vi "Initiate Pulse Test.vi"(7 "Timeout (10000 ms)":u32=10000, 8 "error in":errorcluster, 10 "Tag":u32=1, 11 "VISA resource name":refnum<visa-resource-name>) -> (0 "error out":errorcluster, 1 "Message":string, 2 "Success":bool, 3 "VISA resource name out":refnum<visa-resource-name>, 4 "Command String":string)   [LabVIEW 2012, in "Keithley 2600 Series.lvlib"]
doc: "This VI will instruct the instrument to initiate the output of a pre-configured pulse train.\n\n<b>Functions and Attributes Used</b>\nInititatePulseTest(tag)"
uses:
  Keithley 2600 Series.lvlib
  Private/GlobalVariables.vi
panel:
  # "(c) 2008 Keithley Instruments, Inc.  ALL RIGHTS RESERVED."
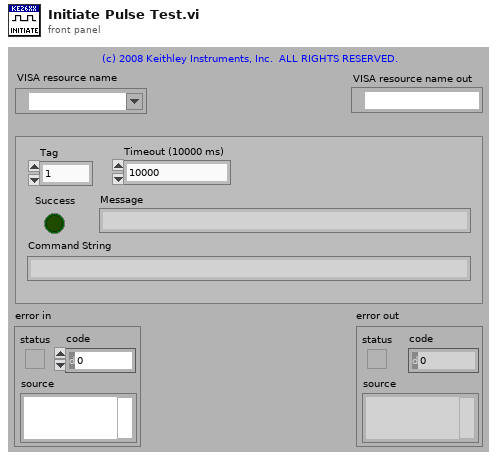
[diagram p1: front panel]
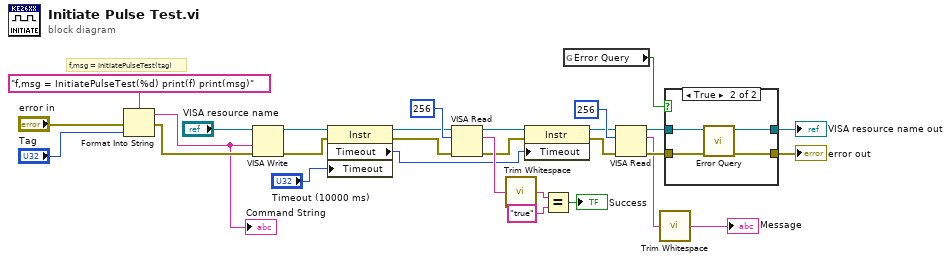
[diagram p0: block diagram]
diagram:
  # "f,msg = InitiatePulseTest(tag)"
  n1 = Format Into String(format string="f,msg = InitiatePulseTest(%d) print(f) print(msg)", error in="error in", "Tag") -> (resulting string=w19:string, error out=w25:errorcluster)  [unwired: 1 in]
  "Command String" <- w19
  n2 = VISA Write(VISA resource name="VISA resource name", write buffer=w19, error in (no error)=w25) -> (VISA resource name out=w10:refnum<visa-resource-name>, error out=w9:errorcluster)  [unwired: 1 out]
  n3 = property class="Instr"(reference=w10, error in=w9, "Timeout"="Timeout (10000 ms)") -> (reference out=w7:refnum<visa-resource-name>, error out=w6:errorcluster, "Timeout"=w5:u32)
  n4 = VISA Read(VISA resource name=w7, byte count=u32 256, error in (no error)=w6) -> (VISA resource name out=w4:refnum<visa-resource-name>, read buffer=w14:string, error out=w3:errorcluster)  [unwired: 1 out]
  n5 = call <vilib>:"Trim Whitespace.vi"("string"=w14) -> ("trimmed string"=w16:string)  [unwired: 1 in]
  n6 = property class="Instr"(reference=w4, error in=w3, "Timeout"=w5) -> (reference out=w2:refnum<visa-resource-name>, error out=w1:errorcluster)
  n7 = Equal?(x=w16, y="true") -> (x = y?=→"Success":bool)
  n8 = global read "GlobalVariables.vi" "Error Query"() -> (w24:bool)
  n9 = VISA Read(VISA resource name=w2, byte count=u32 256, error in (no error)=w1) -> (VISA resource name out=w17:refnum<visa-resource-name>, read buffer=w13:string, error out=w18:errorcluster)  [unwired: 1 out]
  n10 = call <vilib>:"Trim Whitespace.vi"("string"=w13) -> ("trimmed string"=→"Message":string)  [unwired: 1 in]
  n11 = case shown="True" w24 {
    tunnel: [w31 w35] -> w21
    tunnel: [w30 w34] -> w20
    tunnel: w17 -> [w31 w33]
    tunnel: w18 -> [w30 w32]
    frame False {
    }
    frame True {
      n12 = call "Error Query.vi"("error in (no error)"=w32, "VISA resource name"=w33) -> ("error out"=w34:errorcluster, "VISA resource name out"=w35:refnum<visa-resource-name>)  [unwired: 8 out]
    }
  }
  "VISA resource name out" <- w21
  "error out" <- w20
